vi "Read PDF 417 Code.vi"() -> ()   [LabVIEW 2014]
doc: "This example illustrates how to use the Read PDF 417 barcode VI."
uses:
  <vilib>/vision/NI_Vision_Development_Module.lvlib
panel:
  out "Read Time (ms)":dbl format="%.2f"
  out "Data":string
  out "Image":T1(plugin-control)
  # "Overview: Demonstrate the reading PDF 417 barcodes.\nRequirements: Vision Development Module.\nInstructions: Run the VI."
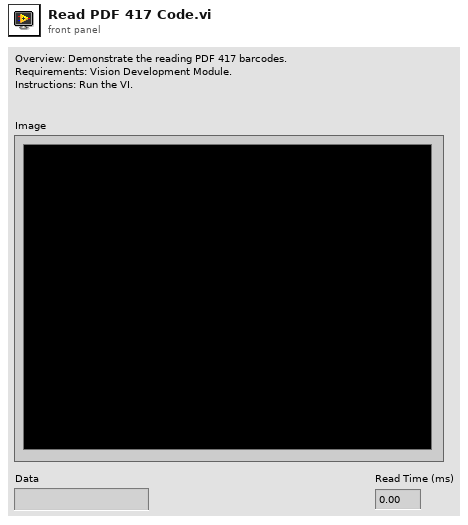
[diagram p1: front panel]
types:
  T1 = typedef "IMAQ Image.ctl" = refnum<image>
  T2 = typedef "Barcode Report" = cluster{"Type":enum32{"PDF417", "Data Matrix ECC 000", "Data Matrix ECC 050", "Data Matrix ECC 080", "Data Matrix ECC 100", "Data Matrix ECC 140", "Data Matrix ECC 200"}, "Binary":bool, "Data":string, "Bounding Box":cluster{"x":sgl, "y":sgl}[], "Errors Corrected":u32, "Erasures Corrected":u32, "Rows":u32, "Columns":u32}
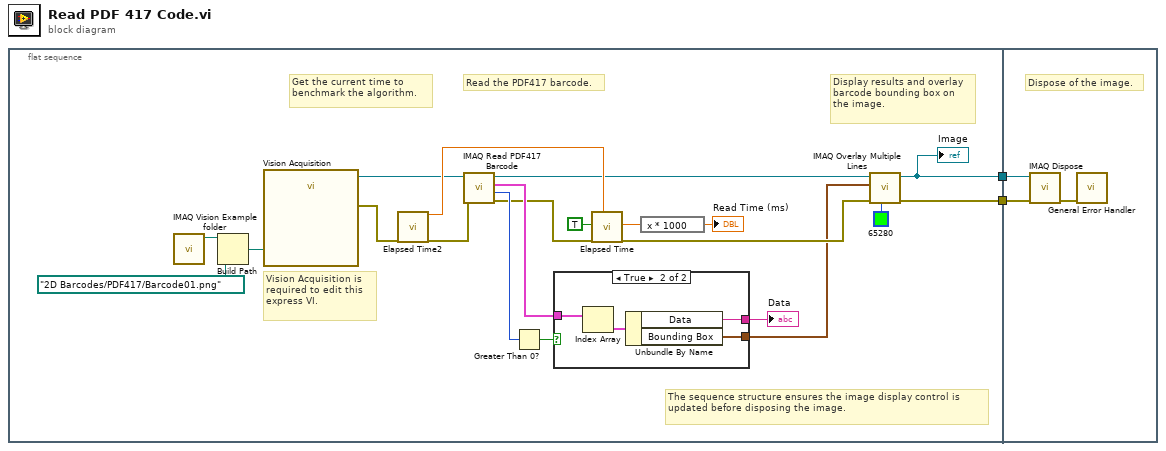
[diagram p0: block diagram]
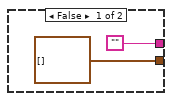
[diagram p2: hidden frame]
diagram:
  n1 = flat-sequence {
    tunnel: [w23] -> w2
    tunnel: [w10] -> w1
    tunnel: w2 -> [w30]
    tunnel: w1 -> [w31]
    frame #0 {
      # "The sequence structure ensures the image display control is updated before disposing the image."
      # "Vision Acquisition is required to edit this express VI."
      # "Read the PDF417 barcode."
      # "Get the current time to benchmark the algorithm."
      # "Display results and overlay barcode bounding box on the image."
      n2 = call "IMAQ Vision Example folder.vi"() -> ("Example Image Path"=w22:path)  [unwired: 11 in]
      n3 = Build Path(base path=w22, name or relative path=path "2D Barcodes/PDF417/Barcode01.png" ("path out")) -> (appended path=w16:path)
      n4 = call "Vision Acquisition"("Image Path"=w16) -> ("Image Out"=w8:T1, "error out"=w18:errorcluster)  [unwired: 25 in]
      n5 = call "Elapsed Time2"("error in (no error)"=w18) -> ("Present (s)"=w14:dbl, "error out"=w9:errorcluster)  [unwired: 11 in, 6 out]
      n6 = call "IMAQ Read PDF417 Barcode"("error in (no error)"=w9, "Image"=w8) -> ("error out"=w6:errorcluster, "Number of Barcodes"=w11:i32, "Barcodes"=w12:T2[], "Image (duplicate)"=w7:T1)  [unwired: 6 in]
      n7 = Greater Than 0?(x=w11) -> (x > 0?=w13:bool)
      n8 = case shown="True" w13 {
        tunnel: w12 -> [_ w29]
        tunnel: [cluster{"x":sgl, "y":sgl}[] [] ("Bounding Box") w27] -> w4
        tunnel: ["" w26] -> w3
        frame False {
        }
        frame True {
          n9 = Index Array(array=w29) -> (element=w28:T2)  [unwired: 1 in]
          n10 = Unbundle By Name(w28) -> ("Data"=w26:string, "Bounding Box"=w27:cluster{"x":sgl, "y":sgl}[])
        }
      }
      "Data" <- w3
      n11 = call "Elapsed Time"("Reset"=TRUE, "error in (no error)"=w6, "Set Start Time (s)"=w14) -> ("Elapsed Time (s)"=w20:dbl, "error out"=w15:errorcluster)  [unwired: 9 in, 6 out]
      n12 = expression code="x * 1000"(w20) -> (→"Read Time (ms)":dbl)
      n13 = call "IMAQ Overlay Multiple Lines"("Color"=u32 65280, "error in (no error)"=w15, "Line End Points"=w4, "Image"=w7) -> ("error out"=w23:errorcluster, "Image Out"=w10:T1)  [unwired: 6 in]
      "Image" <- w10
    }
    frame #1 {
      # "Dispose of the image."
      n14 = call "IMAQ Dispose"("Image"=w31, "error in (no error)"=w30) -> ("error out"=w32:errorcluster)  [unwired: 4 in]
      n15 = call <vilib>:"General Error Handler.vi"("error in (no error)"=w32) -> ()  [unwired: 10 in, 5 out]
    }
  }
